vi "Serial Port - Get Selected Names.vi"(8 "error in (no error)":errorcluster, 11 "Ctrl Refs in":refnum<vi>[](array[refnum])) -> (0 "error out":errorcluster, 1 "Selected Names":string[](array[string]))   [LabVIEW 2011]
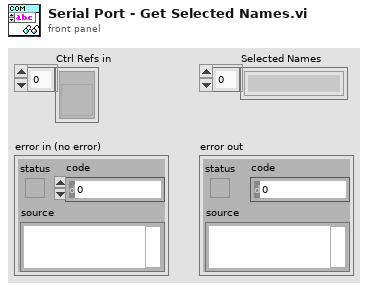
[diagram p1: front panel]
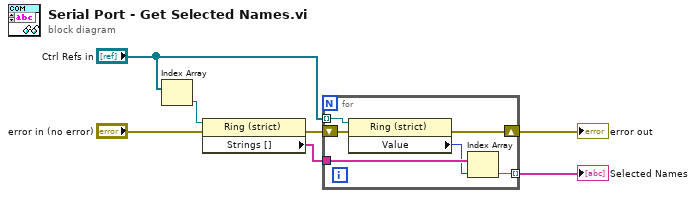
[diagram p0: block diagram]
diagram:
  n1 = Index Array(array="Ctrl Refs in") -> (element=w4:refnum<vi>)  [unwired: 1 in]
  n2 = property class="Ring (strict)"(reference=w4, error in="error in (no error)") -> (error out=w7:errorcluster, "Strings []"=w5:string[])  [unwired: 1 out]
  n3 = for {
    tunnel: "Ctrl Refs in" -> [w13] mode=indexing
    shift-right: [w8] -> w1
    shift-left: w7 -> [w12]
    tunnel: w5 -> [w11]
    tunnel: [w9] -> w2 mode=indexing
    n4 = property class="Ring (strict)"(reference=w13, error in=w12) -> (error out=w8:errorcluster, "Value"=w10:u16)  [unwired: 1 out]
    n5 = Index Array(array=w11, index=w10) -> (element=w9:string)
  }
  "Selected Names" <- w2
  "error out" <- w1
